vi "RequestFIFO6.vi"   [LabVIEW 2016]
uses:
  <vilib>/rvi/Emulation/niFpgaGetClockAttributes.vi
  <vilib>/rvi/Emulation/niFpgaSctlEmulationGetInTimedLoop.vi
  <vilib>/rvi/Emulation/niFpgaEmulationReportErrorSimple.vi
  <vilib>/rvi/interface/RandomDataEmulation/niFpgaRandomDataHandleErrors.vi
  <vilib>/rvi/Emulation/niFpgaEmulationIsFPGAContextNoSignature.vi
  <vilib>/rvi/errors/niFpgaSetErrorForExecOnDevCompSimple.vi
  <vilib>/rvi/eio/common/nirviEmuReportErrorAndStop.vi
  <vilib>/rvi/DataTransferAndStorage/Container/Common/niFpgaContainerGetUniqueNameForEmu.vi
  <vilib>/rvi/FIFO/Fifo_Resource/nirvififoEmulationSetSize.vi
  <vilib>/rvi/FIFO/Fifo_Resource/nirviFifoEmulationQueueMgr.vi
  <instcachedir>/0/nirviFifoEmulationQueueMgr_E5CAEC123FF24DC58D834DCA3CDAA9B5.lvgen/nirviFifoEmulationQueueMgr_E5CAEC123FF24DC58D834DCA3CDAA9B5_005.vi
  <vilib>/Utility/error.llb/Clear Errors.vi
  <vilib>/rvi/FIFO/Fifo_Resource/nirvififoEmulationCreateLock.vi
  <vilib>/rvi/Emulation/niFpgaProcessEmulError.vi
  <vilib>/rvi/FIFO/Fifo_Resource/nirvififoEmulationObtainLock.vi
  <vilib>/rvi/FIFO/Fifo_Resource/nirvififoEmulationReleaseLock.vi
  <vilib>/rvi/occurrence/nirviWaitOnOccurrenceBase.vi
  <vilib>/rvi/errors/nirviReportUnexpectedCaseInternalError.vi
  <vilib>/rvi/errors/nirviReportUnexpectedCaseInternalError (U32).vi
  <instcachedir>/0/nirviFifoEmulationQueueMgr_E5CAEC123FF24DC58D834DCA3CDAA9B5.lvgen/nirviFifoEmulationQueueMgr_E5CAEC123FF24DC58D834DCA3CDAA9B5_007.vi
  <vilib>/rvi/Emulation/niFpgaCriticalErrorInLSC.vi
  <vilib>/rvi/DataTransferAndStorage/Container/XNode/niFpgaContainer.xnode
  <vilib>/rvi/interface/RandomDataEmulation/nirviRandomDataFpgaReadWriteTemplate.vi
  <vilib>/rvi/FIFO/Fifo_Resource/nirvififoEmulationRead.vi
types:
  T1 = typedef "Addresses.ctl" = enum8{"NA", "Accelerometer1X", "Accelerometer1Y", "Accelerometer1Z", "Accelerometer2X", "Accelerometer2Y", "Accelerometer2Z", "Accelerometer3X", "Accelerometer3Y", "Accelerometer3Z", "Accelerometer4X", "Accelerometer4Y", "Accelerometer4Z", "Accelerometer5X", "Accelerometer5Y", "Accelerometer5Z", "Accelerometer6X", "Accelerometer6Y", "Accelerometer6Z", "Sync1", "Sync2", "Sync3", "Sync4", "Accelerometer1", "Accelerometer2", "Accelerometer3", "Accelerometer4", "Accelerometer5", "Accelerometer6", "Accelerometers", "Timestamp", "SamplePeriod"}
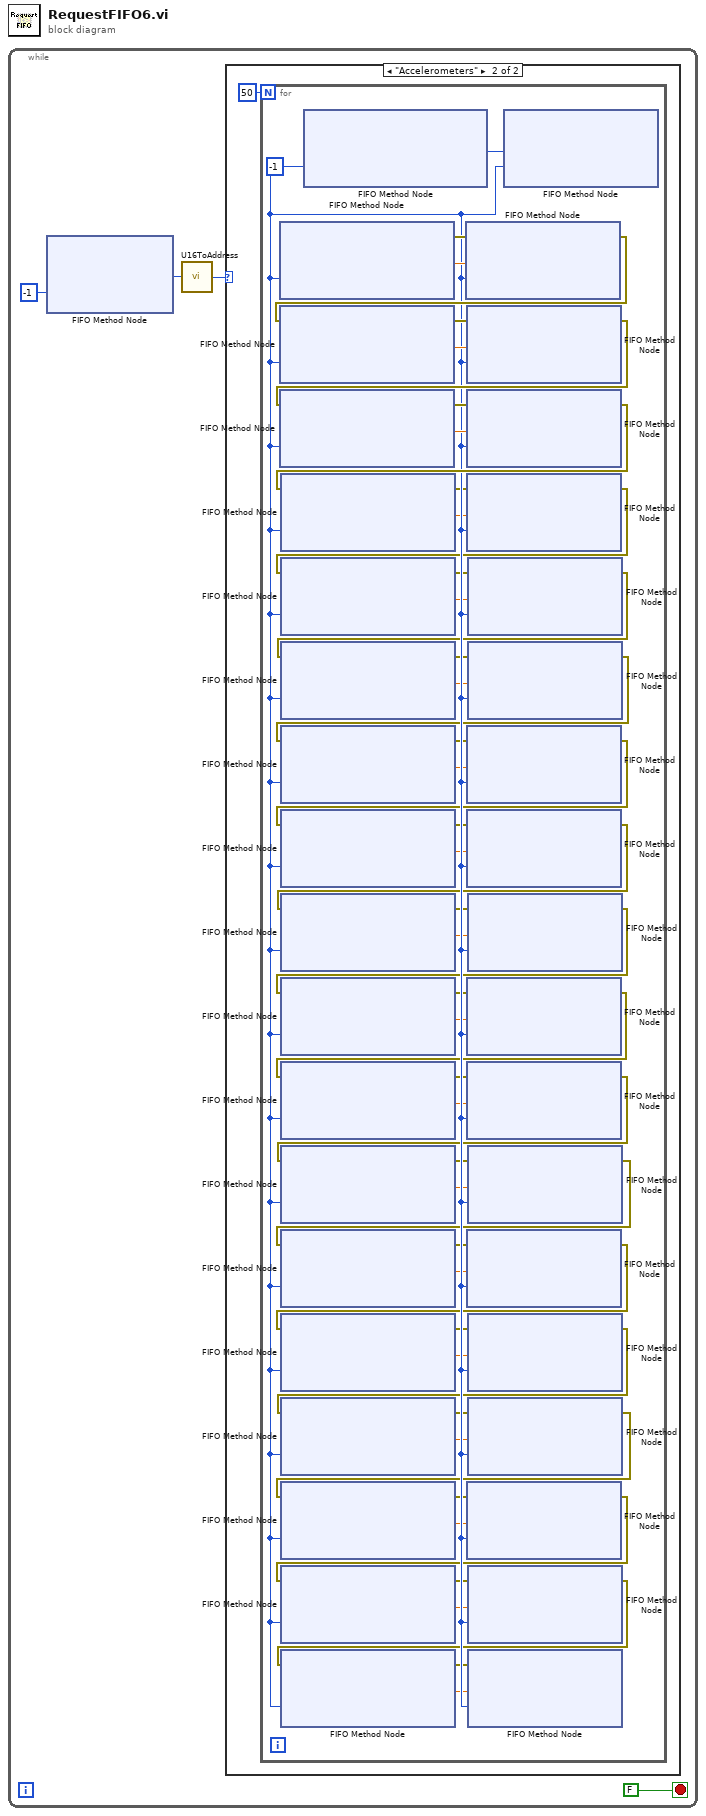
[diagram p0: block diagram]
diagram:
  n1 = while {
    stop <- FALSE stop-if-true
    n2 = xnode ("FIFO Method Node")("Timeout"=-1) -> ("Element"=w2:u16)  [unwired: 1 in, 2 out]
    n3 = call "U16ToAddress.vi"("Input"=w2) -> ("Addresses"=w1:T1)
    n4 = case shown="\"Accelerometers\"" w1 {
      frame "NA", Default {
      }
      frame "Accelerometers" {
        n5 = for {
          N: 50 -> [_]
          w50 = -1 ("Timeout")
          n6 = xnode ("FIFO Method Node")("Timeout"=w50) -> ("Element"=w60:sgl, "error out"=w57:errorcluster)  [unwired: 2 in, 2 out]
          n7 = xnode ("FIFO Method Node")("Timeout"=w50) -> ("Element"=w51:u64)  [unwired: 1 in, 2 out]
          n8 = xnode ("FIFO Method Node")("Element"=w60, "Timeout"=w50, "error in (no error)"=w57) -> ("error out"=w56:errorcluster)  [unwired: 1 in, 2 out]
          n9 = xnode ("FIFO Method Node")("Timeout"=w50, "error in (no error)"=w56) -> ("Element"=w58:sgl, "error out"=w55:errorcluster)  [unwired: 1 in, 2 out]
          n10 = xnode ("FIFO Method Node")("Element"=w58, "Timeout"=w50, "error in (no error)"=w55) -> ("error out"=w54:errorcluster)  [unwired: 1 in, 2 out]
          n11 = xnode ("FIFO Method Node")("Timeout"=w50, "error in (no error)"=w54) -> ("Element"=w59:sgl, "error out"=w53:errorcluster)  [unwired: 1 in, 2 out]
          n12 = xnode ("FIFO Method Node")("Element"=w59, "Timeout"=w50, "error in (no error)"=w53) -> ("error out"=w52:errorcluster)  [unwired: 1 in, 2 out]
          n13 = xnode ("FIFO Method Node")("Timeout"=w50, "error in (no error)"=w52) -> ("Element"=w44:sgl, "error out"=w47:errorcluster)  [unwired: 1 in, 2 out]
          n14 = xnode ("FIFO Method Node")("Element"=w44, "Timeout"=w50, "error in (no error)"=w47) -> ("error out"=w43:errorcluster)  [unwired: 1 in, 2 out]
          n15 = xnode ("FIFO Method Node")("Timeout"=w50, "error in (no error)"=w43) -> ("Element"=w46:sgl, "error out"=w48:errorcluster)  [unwired: 1 in, 2 out]
          n16 = xnode ("FIFO Method Node")("Element"=w46, "Timeout"=w50, "error in (no error)"=w48) -> ("error out"=w42:errorcluster)  [unwired: 1 in, 2 out]
          n17 = xnode ("FIFO Method Node")("Timeout"=w50, "error in (no error)"=w42) -> ("Element"=w45:sgl, "error out"=w49:errorcluster)  [unwired: 1 in, 2 out]
          n18 = xnode ("FIFO Method Node")("Element"=w45, "Timeout"=w50, "error in (no error)"=w49) -> ("error out"=w33:errorcluster)  [unwired: 1 in, 2 out]
          n19 = xnode ("FIFO Method Node")("Timeout"=w50, "error in (no error)"=w33) -> ("Element"=w39:sgl, "error out"=w36:errorcluster)  [unwired: 1 in, 2 out]
          n20 = xnode ("FIFO Method Node")("Element"=w39, "Timeout"=w50, "error in (no error)"=w36) -> ("error out"=w40:errorcluster)  [unwired: 1 in, 2 out]
          n21 = xnode ("FIFO Method Node")("Timeout"=w50, "error in (no error)"=w40) -> ("Element"=w37:sgl, "error out"=w35:errorcluster)  [unwired: 1 in, 2 out]
          n22 = xnode ("FIFO Method Node")("Element"=w37, "Timeout"=w50, "error in (no error)"=w35) -> ("error out"=w41:errorcluster)  [unwired: 1 in, 2 out]
          n23 = xnode ("FIFO Method Node")("Timeout"=w50, "error in (no error)"=w41) -> ("Element"=w38:sgl, "error out"=w34:errorcluster)  [unwired: 1 in, 2 out]
          n24 = xnode ("FIFO Method Node")("Element"=w38, "Timeout"=w50, "error in (no error)"=w34) -> ("error out"=w24:errorcluster)  [unwired: 1 in, 2 out]
          n25 = xnode ("FIFO Method Node")("Timeout"=w50, "error in (no error)"=w24) -> ("Element"=w27:sgl, "error out"=w30:errorcluster)  [unwired: 1 in, 2 out]
          n26 = xnode ("FIFO Method Node")("Element"=w27, "Timeout"=w50, "error in (no error)"=w30) -> ("error out"=w26:errorcluster)  [unwired: 1 in, 2 out]
          n27 = xnode ("FIFO Method Node")("Timeout"=w50, "error in (no error)"=w26) -> ("Element"=w29:sgl, "error out"=w31:errorcluster)  [unwired: 1 in, 2 out]
          n28 = xnode ("FIFO Method Node")("Element"=w29, "Timeout"=w50, "error in (no error)"=w31) -> ("error out"=w25:errorcluster)  [unwired: 1 in, 2 out]
          n29 = xnode ("FIFO Method Node")("Timeout"=w50, "error in (no error)"=w25) -> ("Element"=w28:sgl, "error out"=w32:errorcluster)  [unwired: 1 in, 2 out]
          n30 = xnode ("FIFO Method Node")("Element"=w28, "Timeout"=w50, "error in (no error)"=w32) -> ("error out"=w15:errorcluster)  [unwired: 1 in, 2 out]
          n31 = xnode ("FIFO Method Node")("Timeout"=w50, "error in (no error)"=w15) -> ("Element"=w21:sgl, "error out"=w18:errorcluster)  [unwired: 1 in, 2 out]
          n32 = xnode ("FIFO Method Node")("Element"=w21, "Timeout"=w50, "error in (no error)"=w18) -> ("error out"=w22:errorcluster)  [unwired: 1 in, 2 out]
          n33 = xnode ("FIFO Method Node")("Timeout"=w50, "error in (no error)"=w22) -> ("Element"=w19:sgl, "error out"=w17:errorcluster)  [unwired: 1 in, 2 out]
          n34 = xnode ("FIFO Method Node")("Element"=w19, "Timeout"=w50, "error in (no error)"=w17) -> ("error out"=w23:errorcluster)  [unwired: 1 in, 2 out]
          n35 = xnode ("FIFO Method Node")("Timeout"=w50, "error in (no error)"=w23) -> ("Element"=w20:sgl, "error out"=w16:errorcluster)  [unwired: 1 in, 2 out]
          n36 = xnode ("FIFO Method Node")("Element"=w20, "Timeout"=w50, "error in (no error)"=w16) -> ("error out"=w6:errorcluster)  [unwired: 1 in, 2 out]
          n37 = xnode ("FIFO Method Node")("Timeout"=w50, "error in (no error)"=w6) -> ("Element"=w9:sgl, "error out"=w12:errorcluster)  [unwired: 1 in, 2 out]
          n38 = xnode ("FIFO Method Node")("Element"=w9, "Timeout"=w50, "error in (no error)"=w12) -> ("error out"=w8:errorcluster)  [unwired: 1 in, 2 out]
          n39 = xnode ("FIFO Method Node")("Timeout"=w50, "error in (no error)"=w8) -> ("Element"=w11:sgl, "error out"=w13:errorcluster)  [unwired: 1 in, 2 out]
          n40 = xnode ("FIFO Method Node")("Element"=w11, "Timeout"=w50, "error in (no error)"=w13) -> ("error out"=w7:errorcluster)  [unwired: 1 in, 2 out]
          n41 = xnode ("FIFO Method Node")("Timeout"=w50, "error in (no error)"=w7) -> ("Element"=w10:sgl, "error out"=w14:errorcluster)  [unwired: 1 in, 2 out]
          n42 = xnode ("FIFO Method Node")("Element"=w10, "Timeout"=w50, "error in (no error)"=w14) -> ()  [unwired: 1 in, 3 out]
          n43 = xnode ("FIFO Method Node")("Element"=w51, "Timeout"=w50) -> ()  [unwired: 1 in, 2 out]
        }
      }
    }
  }
